vi "Get json value after prefix.vi"(8 "error in (no error)":errorcluster, 10 "Token prefix":string, 11 "String in":string) -> (0 "error out":errorcluster, 3 "String after prefix to EOL":string)   [LabVIEW 2013]
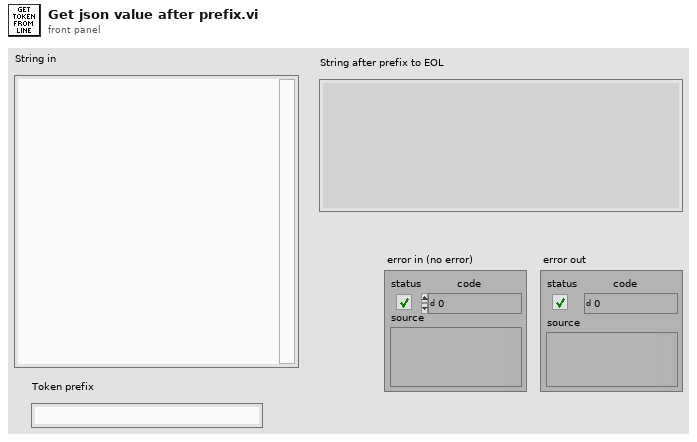
[diagram p1: front panel]
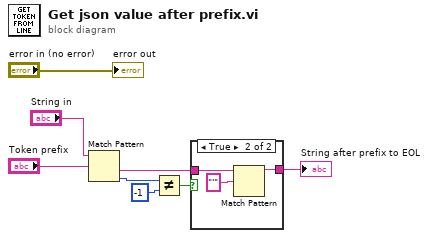
[diagram p0: block diagram]
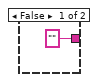
[diagram p2: hidden frame]
diagram:
  n1 = Match Pattern(string="String in", regular expression="Token prefix") -> (after substring=w7:string, offset past match=w4:i32)  [unwired: 1 in, 2 out]
  n2 = Not Equal?(x=w4, y=-1) -> (x != y?=w6:bool)
  n3 = case shown="True" w6 {
    tunnel: w7 -> [_ w12]
    tunnel: ["" ("read buffer") w10] -> w8
    frame False {
    }
    frame True {
      n4 = Match Pattern(string=w12, regular expression="'") -> (before substring=w10:string)  [unwired: 1 in, 3 out]
    }
  }
  "String after prefix to EOL" <- w8
  "error out" <- "error in (no error)"
